vi "random between.vi"(8 "min":dbl, 9 "max":dbl) -> (1 "x+y":i32)   [LabVIEW 2014]
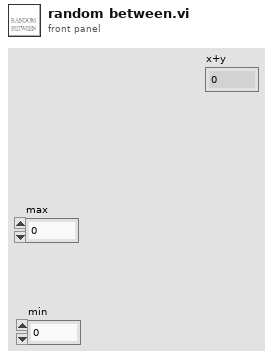
[diagram p1: front panel]
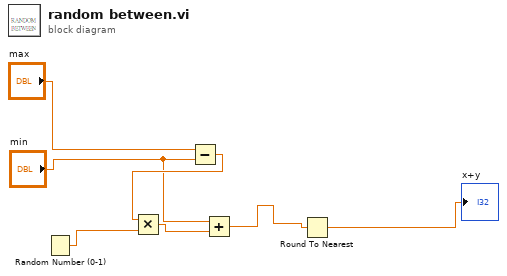
[diagram p0: block diagram]
diagram:
  n1 = Random Number (0-1)() -> (number: 0 to 1=w6:dbl)
  n2 = Subtract(x="max", y="min") -> (x-y=w5:dbl)
  n3 = Multiply(x=w5, y=w6) -> (x*y=w3:dbl)
  n4 = Add(x="min", y=w3) -> (x+y=w2:dbl)
  n5 = Round To Nearest(number=w2) -> (nearest integer value=→"x+y":dbl)
